vi "Switch Configuration - Topology Data.vi"(8 "error in (no error)":errorcluster, 10 "Mux Topology":string(combo)="2503/2-Wire 24x1 Mux" caption="Topology") -> (0 "error out":errorcluster, 1 "Topology Data":T1)   [LabVIEW 2015, in "DMM-SWITCH-ScanList System Explorer.lvlib"]
doc: "Extract Mux Topology relevant data from the selected Mux Topology string."
uses:
  DMM-SWITCH-ScanList System Explorer.lvlib
  Configuration Controls/Topology Data.ctl
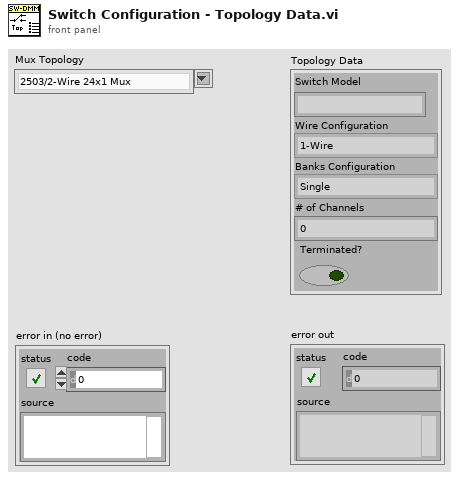
[diagram p1: front panel]
types:
  T1 = typedef "DMM-SWITCH-ScanList System Explorer.lvlib/Topology Data.ctl" = cluster{"Switch Model":string, "Wire Configuration":enum16{"1-Wire", "2-Wire", "4-Wire"}, "Banks Configuration":enum16{"Single", "Dual", "Quad", "Octal", "Sixteen"}, "# of Channels":u32, "Terminated?":bool}
  T2 = enum16{"Single", "Dual", "Quad", "Octal", "Sixteen"}
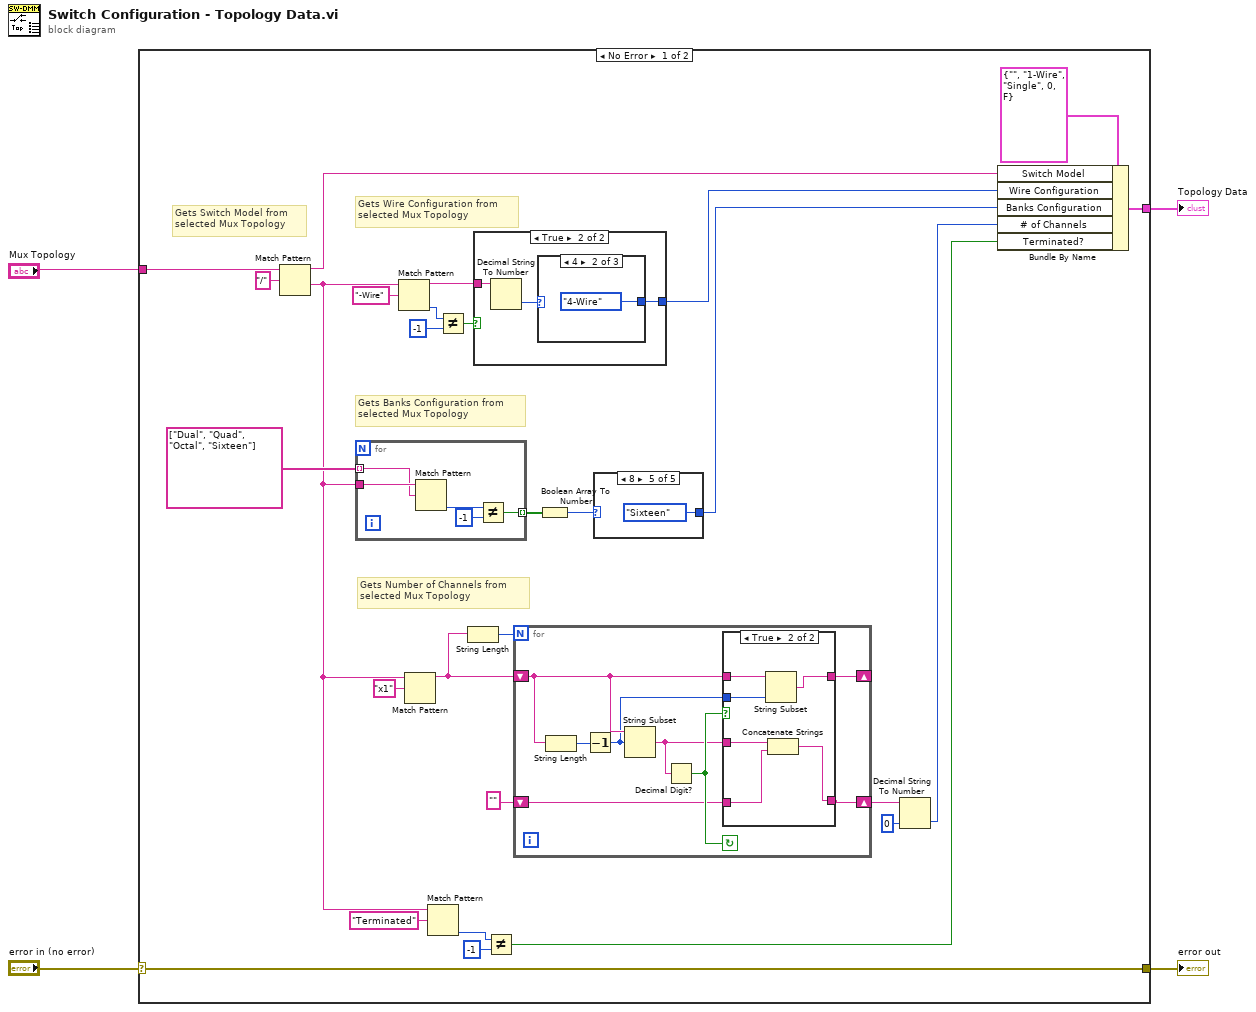
[diagram p0: block diagram]
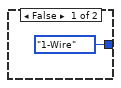
[diagram p2: hidden frame]
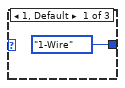
[diagram p3: hidden frame]
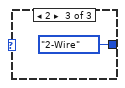
[diagram p4: hidden frame]
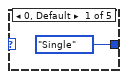
[diagram p6: hidden frame]
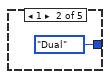
[diagram p7: hidden frame]
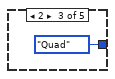
[diagram p8: hidden frame]
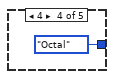
[diagram p9: hidden frame]
diagram:
  n1 = case shown="No Error" "error in (no error)" {
    selector: "error in (no error)" -> [w13 w66]
    tunnel: "Mux Topology" -> [w32 _]
    tunnel: [w25 _] -> w3
    tunnel: [w13 w66] -> w1
    frame No Error {
      # "Gets Banks Configuration from \nselected Mux Topology"
      # "Gets Number of Channels from \nselected Mux Topology"
      # "Gets Wire Configuration from \nselected Mux Topology"
      # "Gets Switch Model from \nselected Mux Topology"
      n2 = Match Pattern(string=w32, regular expression="/") -> (before substring=w21:string, after substring=w12:string)  [unwired: 1 in, 2 out]
      n3 = for {
        tunnel: string[] ["Dual", "Quad", "Octal", "Sixteen"] ("Array") -> [w62] mode=indexing
        tunnel: w12 -> [w63]
        tunnel: [w61] -> w28 mode=indexing
        n4 = Match Pattern(string=w63, regular expression=w62) -> (offset past match=w64:i32)  [unwired: 1 in, 3 out]
        n5 = Not Equal?(x=w64, y=-1) -> (x != y?=w61:bool)
      }
      n6 = Match Pattern(string=w12, regular expression="-Wire") -> (before substring=w18:string, offset past match=w7:i32)  [unwired: 1 in, 2 out]
      n7 = Match Pattern(string=w12, regular expression="x1") -> (before substring=w19:string)  [unwired: 1 in, 3 out]
      n8 = Match Pattern(string=w12, regular expression="Terminated") -> (offset past match=w9:i32)  [unwired: 1 in, 3 out]
      n9 = Not Equal?(x=w7, y=-1) -> (x != y?=w5:bool)
      n10 = String Length(string=w19) -> (length=w23:i32)
      n11 = case shown="True" w5 {
        tunnel: w18 -> [_ w36]
        tunnel: [enum16{"1-Wire", "2-Wire", "4-Wire"}."1-Wire" ("Wire Configuration") w34] -> w17
        frame False {
        }
        frame True {
          n12 = Decimal String To Number(string=w36) -> (number=w35:i32)  [unwired: 2 in, 1 out]
          n13 = case shown="4" w35 {
            tunnel: [enum16{"1-Wire", "2-Wire", "4-Wire"}."1-Wire" ("Wire Configuration") enum16{"1-Wire", "2-Wire", "4-Wire"}."4-Wire" ("Wire Configuration") enum16{"1-Wire", "2-Wire", "4-Wire"}."2-Wire" ("Wire Configuration")] -> w34
            frame 1, Default {
            }
            frame 4 {
            }
            frame 2 {
            }
          }
        }
      }
      n14 = Not Equal?(x=w9, y=-1) -> (x != y?=w8:bool)
      n15 = for {
        N: w23 -> [_]
        shift-right: [w44] -> _
        shift-left: w19 -> [w46]
        shift-right: [w40] -> w16
        shift-left: "" -> [w42]
        stop <- w43 continue-if-true
        n16 = String Length(string=w46) -> (length=w47:i32)
        n17 = Decrement(x=w47) -> (x-1=w45:i32)
        n18 = String Subset(string=w46, offset (0)=w45) -> (substring=w41:string)  [unwired: 1 in]
        n19 = Decimal Digit?(1:w41) -> (0:w43:bool)
        n20 = case shown="True" w43 {
          tunnel: w46 -> [w49 w55]
          tunnel: w45 -> [_ w53]
          tunnel: [w49 w54] -> w44
          tunnel: w42 -> [w48 w50]
          tunnel: w41 -> [_ w51]
          tunnel: [w48 w52] -> w40
          frame False {
          }
          frame True {
            n21 = String Subset(string=w55, length (rest)=w53) -> (substring=w54:string)  [unwired: 1 in]
            n22 = Concatenate Strings(w51, w50) -> (w52:string)
          }
        }
      }
      n23 = Boolean Array To Number(Boolean array=w28) -> (number=w27:u32)
      n24 = case shown="8" w27 {
        tunnel: [T2."Single" ("Banks Configuration") T2."Dual" ("Banks Configuration") T2."Quad" ("Banks Configuration") T2."Octal" ("Banks Configuration") T2."Sixteen" ("Banks Configuration")] -> w26
        frame 0, Default {
        }
        frame 1 {
        }
        frame 2 {
        }
        frame 4 {
        }
        frame 8 {
        }
      }
      n25 = Decimal String To Number(string=w16, default (0L)=u32 0 ("default (0 I32)")) -> (number=w15:u32)  [unwired: 1 in, 1 out]
      n26 = Bundle By Name(cluster=T1 {"Switch Model"="", "Wire Configuration"=enum."1-Wire", "Banks Configuration"=enum."Single", "# of Channels"=0, "Terminated?"=FALSE} ("Topology Data"), "Switch Model"=w21, "Wire Configuration"=w17, "Banks Configuration"=w26, "# of Channels"=w15, "Terminated?"=w8) -> (w25:T1)
    }
    frame Error {
    }
  }
  "Topology Data" <- w3
  "error out" <- w1
